vi "galvoWriteClose.vi"   [LabVIEW 2017]
uses:
  globalDevices.vi
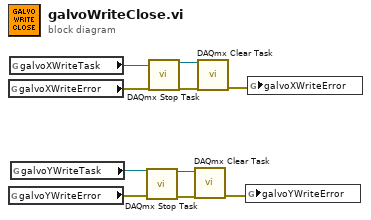
[diagram p0: block diagram]
diagram:
  n1 = global read "globalDevices.vi" "galvoXWriteError"() -> (w9:errorcluster)
  n2 = global read "globalDevices.vi" "galvoYWriteError"() -> (w7:errorcluster)
  n3 = global read "globalDevices.vi" "galvoXWriteTask"() -> (w10:refnum<k21>)
  n4 = global read "globalDevices.vi" "galvoYWriteTask"() -> (w8:refnum<k21>)
  n5 = call <vilib>:"DAQmx Stop Task.vi"("task/channels in"=w8, "error in"=w7) -> ("task out"=w4:refnum<k21>, "error out"=w3:errorcluster)  [unwired: 12 in]
  n6 = call <vilib>:"DAQmx Stop Task.vi"("task/channels in"=w10, "error in"=w9) -> ("task out"=w6:refnum<k21>, "error out"=w5:errorcluster)  [unwired: 12 in]
  n7 = call <vilib>:"DAQmx Clear Task.vi"("task in"=w4, "error in"=w3) -> ("error out"=w1:errorcluster)  [unwired: 13 in]
  n8 = call <vilib>:"DAQmx Clear Task.vi"("task in"=w6, "error in"=w5) -> ("error out"=w2:errorcluster)  [unwired: 13 in]
  n9 = global write "globalDevices.vi" "galvoYWriteError"(w1) -> ()
  n10 = global write "globalDevices.vi" "galvoXWriteError"(w2) -> ()
